vi "Check Graph Validity.vi"(8 "error in (no error)":errorcluster, 11 "Live Graph Plotter in":refnum<class "Live Graph Plotter.lvclass">) -> (0 "error out":errorcluster, 3 "Live Graph Plotter out":refnum<class "Live Graph Plotter.lvclass">)   [LabVIEW 2025, in "Live Graph Plotter.lvclass"]
doc: "Check if the waveform graph ref is initialized. If not, throw error."
uses:
  Live Graph Plotter.lvclass
  Live Graph Plotter.lvclass/Live Graph Plotter.ctl
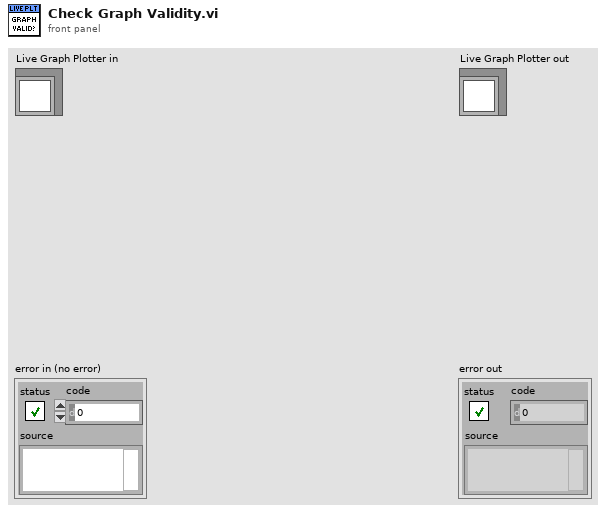
[diagram p1: front panel]
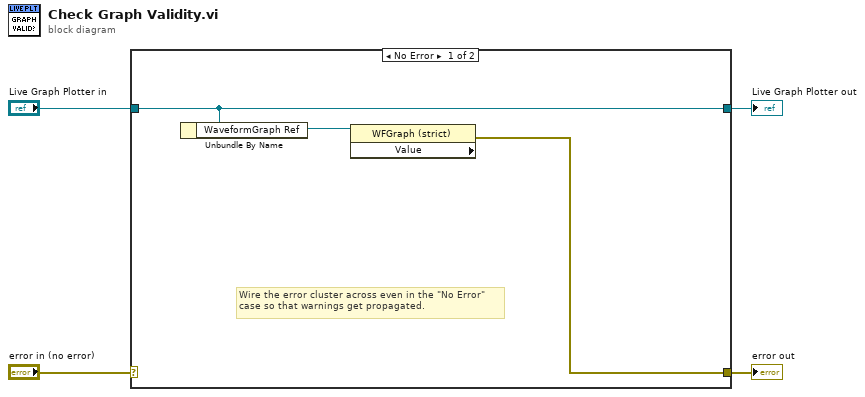
[diagram p0: block diagram]
diagram:
  n1 = case shown="No Error" "error in (no error)" {
    selector: "error in (no error)" -> [_ w9]
    tunnel: [w5 w9] -> w3
    tunnel: [w7 w8] -> w1
    tunnel: "Live Graph Plotter in" -> [w7 w8]
    frame No Error {
      # "Wire the error cluster across even in the \"No Error\"\ncase so that warnings get propagated."
      n2 = Unbundle By Name(w7) -> ("WaveformGraph Ref"=w6:refnum<vi>)
      n3 = property class="WFGraph (strict)" props=["Value"](reference=w6) -> (error out=w5:errorcluster)  [unwired: 1 in, 2 out]
    }
    frame Error {
    }
  }
  "error out" <- w3
  "Live Graph Plotter out" <- w1
